vi "populateHardpointActuatorSteps.vi"(8 "error in (no error)":errorcluster, 10 "Steps":i16[](array[numeric]), 11 "Model in":refnum<class "Model.lvclass">) -> (0 "error out":errorcluster, 3 "Model out":refnum<class "Model.lvclass">)   [LabVIEW 2016, in "Model.lvclass"]
uses:
  Model.lvclass
  Model.lvclass/Model.ctl
  ILCCommunications/ILCCommunications.lvclass/ILCCommunications.ctl
  Common_RT_HPILC/HPILC/HPILC.lvclass/HPILC.ctl
  ILCCommunications/ILCCommunications.lvclass
  Common_RT_HPILC/HPILC/HPILC.lvclass
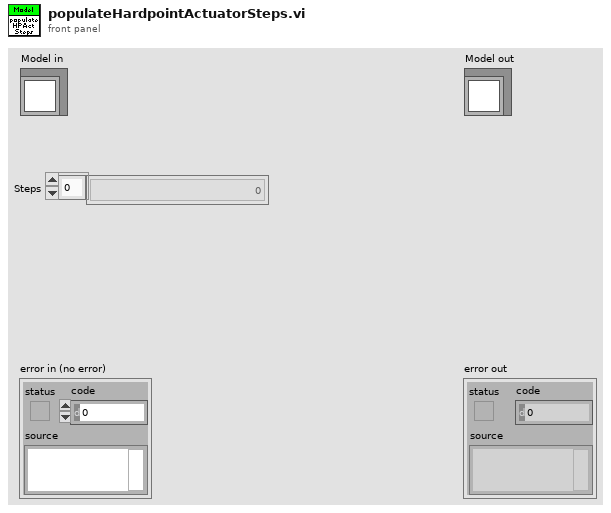
[diagram p1: front panel]
types:
  T1 = typedef "RTHPILC.lvlib/HPData.ctl" = cluster{"Constants":T2, "Command":T3, "Telemetry":T4, "Responses":T5, "Timings":T7}
  T2 = typedef "RTHPILC.lvlib/HPConstants.ctl" = cluster{"ID":i16, "ReferencePosition":i32, "XPosition":sgl, "YPosition":sgl, "ZPosition":sgl}
  T3 = typedef "RTHPILC.lvlib/HPCommand.ctl" = cluster{"Steps":i8}
  T4 = typedef "RTHPILC.lvlib/HPTelemetry.ctl" = cluster{"ILCFault":bool, "LimitSwitchCWOperated":bool, "LimitSwitchCCWOperated":bool, "BroadcastCounter":u8, "SSIEncoderValue":i32, "LoadCellForce":sgl}
  T5 = typedef "RTHPILC.lvlib/HPResponses.ctl" = cluster{"StepMotor":T6, "ForceAndStatus":T6}
  T6 = typedef "RTModbus.lvlib/ExceptionCodes.ctl" = u16
  T7 = typedef "RTHPILC.lvlib/HPTimings.ctl" = cluster{"BroadcastStepMotor":u32, "ForceAndStatus":u32, "FreezeSensorValues":u32, "StepMotor":u32}
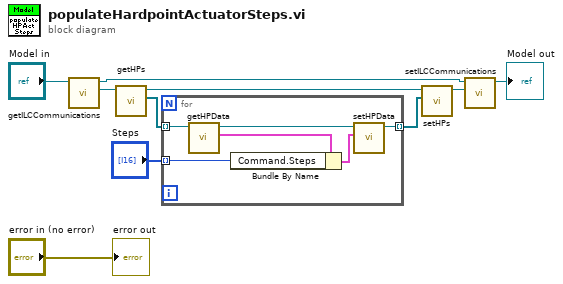
[diagram p0: block diagram]
diagram:
  n1 = call "getILCCommunications.vi"("Model in"="Model in") -> ("ILCCommunications"=w5:refnum<class "ILCCommunications.lvclass">, "Model out"=w4:refnum<class "Model.lvclass">)  [unwired: 9 in]
  n2 = call "getHPs.vi"("ILCCommunications in"=w5) -> ("HPs"=w10:refnum<class "HPILC.lvclass">[], "ILCCommunications out"=w7:refnum<class "ILCCommunications.lvclass">)  [unwired: 9 in]
  n3 = for {
    tunnel: w10 -> [w16] mode=indexing
    tunnel: [w14] -> w9 mode=indexing
    tunnel: "Steps" -> [w11] mode=indexing
    n4 = call "getHPData.vi"("HPILC in"=w16) -> ("HPData"=w13:T1, "HPILC out"=w15:refnum<class "HPILC.lvclass">)  [unwired: 9 in]
    n5 = Bundle By Name(cluster=w13, "Command.Steps"=w11) -> (w12:T1)
    n6 = call "setHPData.vi"("HPData"=w12, "HPILC in"=w15) -> ("HPILC out"=w14:refnum<class "HPILC.lvclass">)  [unwired: 9 in]
  }
  n7 = call "setHPs.vi"("HPs"=w9, "ILCCommunications in"=w7) -> ("ILCCommunications out"=w6:refnum<class "ILCCommunications.lvclass">)  [unwired: 9 in]
  n8 = call "setILCCommunications.vi"("ILCCommunications"=w6, "Model in"=w4) -> ("Model out"=→"Model out":refnum<class "Model.lvclass">)  [unwired: 9 in]
  "error out" <- "error in (no error)"
